vi "Get PanelArray.vi"(8 "error in (no error)":errorcluster, 11 "AppListPanel in":refnum<class "AppListPanel.lvclass">) -> (0 "error out":errorcluster, 2 "PanelArray":refnum<class "ArrayManager.lvclass">, 3 "AppListPanel out":refnum<class "AppListPanel.lvclass">)   [LabVIEW 2020, in "PicoG-App.lvlib" / "AppListPanel.lvclass"]
uses:
  AppListPanel.lvclass
  <vilib>/IlluminatedG/IG OOPanel/OOPanel/ArrayManager/ArrayManager.lvclass
  AppListPanel.lvclass/AppListPanel.ctl
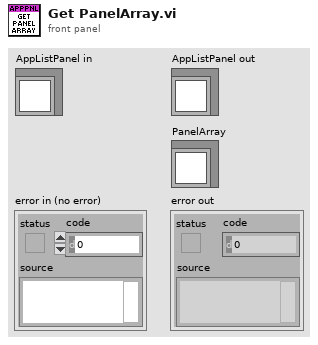
[diagram p1: front panel]
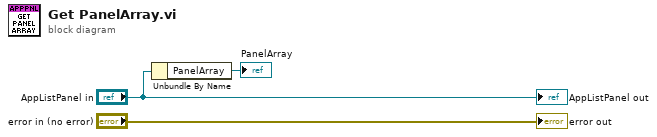
[diagram p0: block diagram]
diagram:
  n1 = Unbundle By Name("AppListPanel in") -> ("PanelArray"=→"PanelArray":refnum<class "ArrayManager.lvclass">)
  "error out" <- "error in (no error)"
  "AppListPanel out" <- "AppListPanel in"
